vi "C-R Speed Test AIN eAddresses.vi"() -> ()   [LabVIEW 2020]
panel:
  in  "Case Constant\n(See Context Help)":bool
  out "Sorted Interval Array":ext[](array[numeric]) format="%.3g"
  in  "Range":dbl=10.0 format="%.2f"
  out "ConnectionType Out":i32
  out "DeviceType Out":i32
  in  "Identifier":string="LJM_idANY"
  in  "ConnectionType":string="LJM_ctANY"
  in  "DeviceType":string="LJM_dtANY"
  in  "Enable Interval Timing":bool
  out "min ms":ext format="%.3g"
  out "max ms":ext format="%.3g"
  out "avg ms per iteration":ext format="%.3f"
  out "Interval Array":ext[](array[numeric]) format="%.3g"
  in  "Write Both DACs":bool
  in  "Write Digital":bool
  in  "Read Digital":bool
  out "total ms":ext format="%.3g"
  in  "# Iterations":i32=1000
  in  "# AIN Channels":i32=1
  in  "Settling":i32
  out "Error Message":string
  in  "Resolution Index":i32=1
  out "error out":errorcluster
  # "Set controls as desired then click arrow (upper-left of window) to run.\n\nThis version uses a call before the loop to convert all names to addresses, and then inside the loop it uses a single call to eAddresses for all writes & reads."
  # "Interval timing uses the high resolution GetHostTick\nfunction from the LJM library."
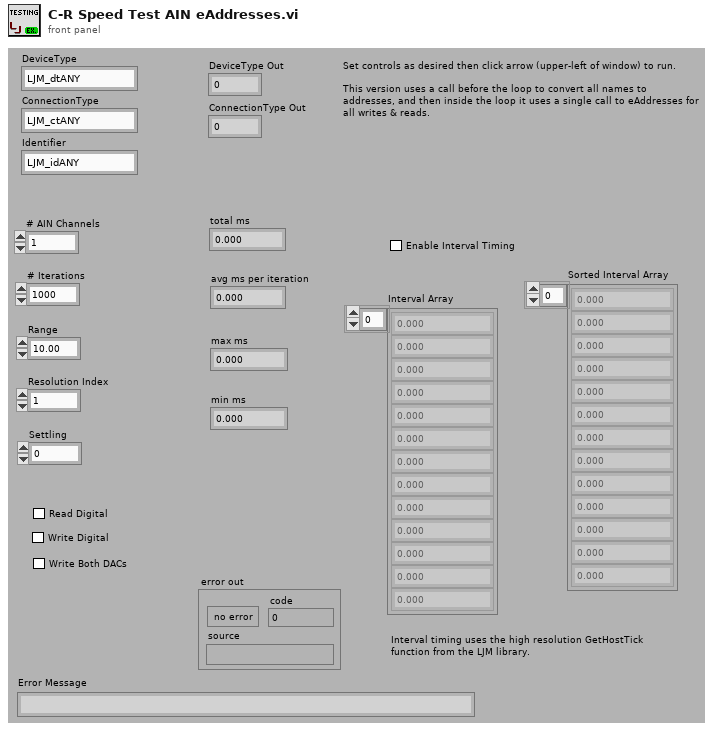
[diagram p1: front panel]
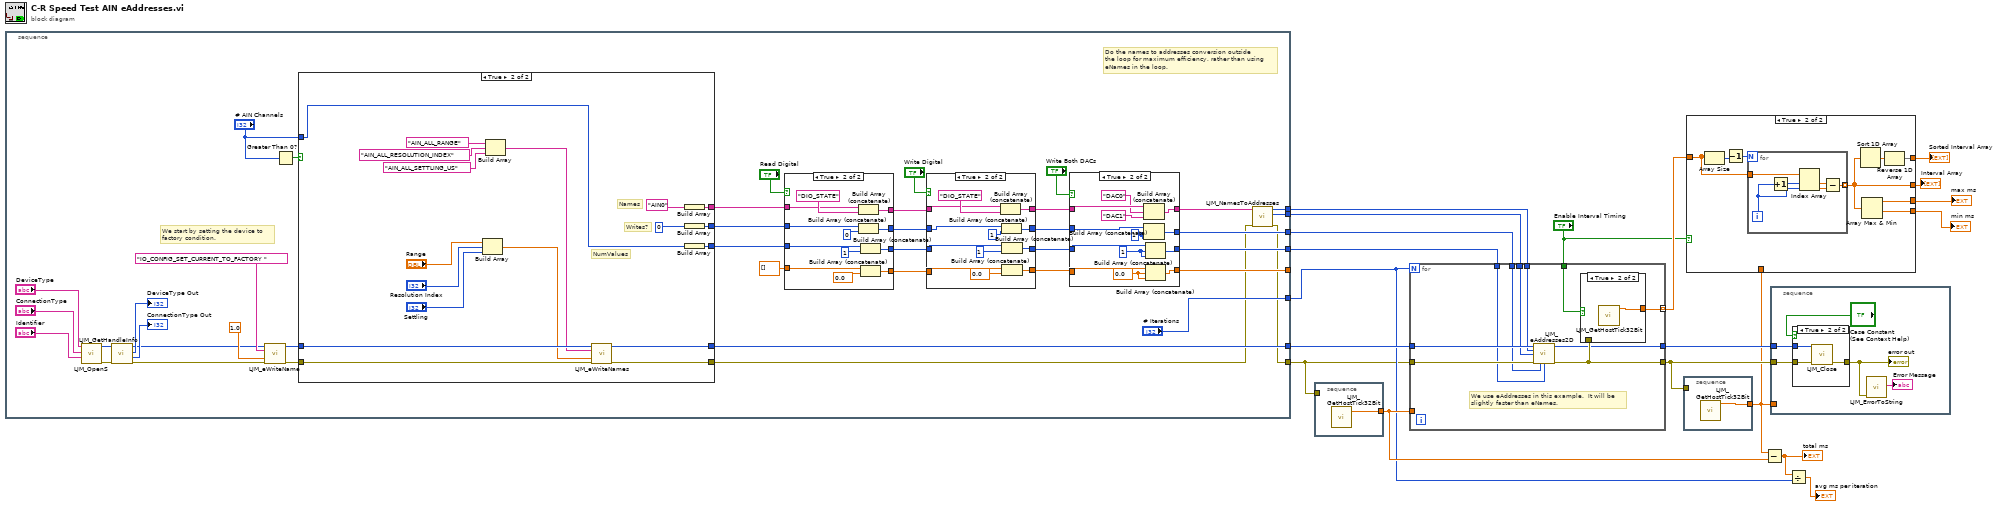
[diagram p0: block diagram]
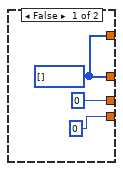
[diagram p2: hidden frame]
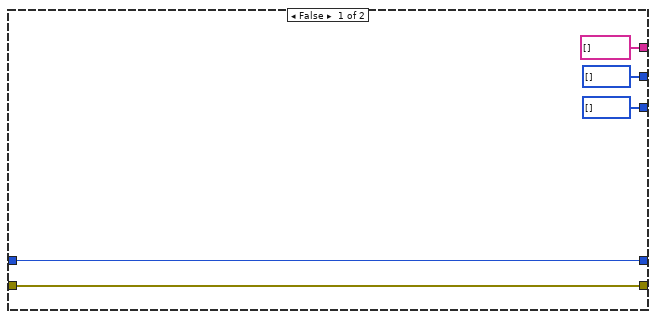
[diagram p4: hidden frame]
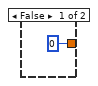
[diagram p8: hidden frame]
diagram:
  n1 = stacked-sequence {
    tunnel: [w40] -> w19
    tunnel: [w26] -> w2
    tunnel: ["# Iterations"] -> w14
    tunnel: [w29] -> w4
    tunnel: [w33] -> w10
    tunnel: [w32] -> w9
    tunnel: [w31] -> _
    tunnel: [w28] -> w3
    frame #0 {
      # "We start by setting the device to\nfactory condition."
      # "Do the names to addresses conversion outside\nthe loop for maximum efficiency, rather than using\neNames in the loop."
      n2 = call "LJM_OpenS.vi"("Identifier"="Identifier", "ConnectionType"="ConnectionType", "DeviceType"="DeviceType") -> ("error out"=w45:errorcluster, "Handle"=w46:i32)  [unwired: 7 in]
      n3 = call "LJM_GetHandleInfo.vi"("error in"=w45, "Handle In"=w46) -> ("error out"=w24:errorcluster, "ConnectionType"=→"ConnectionType Out":i32, "DeviceType"=→"DeviceType Out":i32, "Handle Out"=w21:i32)  [unwired: 2 in, 4 out]
      n4 = call "LJM_eWriteName.vi"("Handle In"=w21, "Name"="IO_CONFIG_SET_CURRENT_TO_FACTORY ", "Value"=1.0, "error in"=w24) -> ("Handle Out"=w20:i32, "error out"=w23:errorcluster)  [unwired: 10 in]
      n5 = Greater Than 0?(x="# AIN Channels") -> (x > 0?=w42:bool)
      n6 = case shown="True" w42 {
        tunnel: "# AIN Channels" -> [_ w72]
        tunnel: w20 -> [w64 w82]
        tunnel: w23 -> [w63 w81]
        tunnel: [w63 w80] -> w27
        tunnel: [w64 w79] -> w40
        tunnel: [string[] [] w74] -> w39
        tunnel: [i32[] [] w73] -> w38
        tunnel: [i32[] [] w71] -> w36
        frame False {
        }
        frame True {
          # "NumValues"
          # "Names"
          # "Writes?"
          n7 = Build Array("Range", "Resolution Index", "Settling") -> (w78:dbl[])
          n8 = Build Array("AIN_ALL_RANGE" ("Substring"), "AIN_ALL_RESOLUTION_INDEX" ("Substring"), "AIN_ALL_SETTLING_US" ("Substring")) -> (w77:string[])
          n9 = call "LJM_eWriteNames.vi"("Handle In"=w82, "aNames"=w77, "aValuesIn"=w78, "error in"=w81) -> ("Handle Out"=w79:i32, "error out"=w80:errorcluster)  [unwired: 9 in, 1 out]
          n10 = Build Array("AIN0") -> (w74:string[])
          n11 = Build Array(0) -> (w73:i32[])
          n12 = Build Array(w72) -> (w71:i32[])
        }
      }
      n13 = case shown="True" "Read Digital" {
        tunnel: [w119 w126] -> w57
        tunnel: [w117 w128] -> w56
        tunnel: [w116 w127] -> w55
        tunnel: w39 -> [w119 w125]
        tunnel: w38 -> [w118 w124]
        tunnel: dbl[] [] ("Input Array") -> [w116 w123]
        tunnel: w36 -> [w117 w122]
        tunnel: [w118 w121] -> w35
        frame False {
        }
        frame True {
          n14 = Build Array (concatenate)(w125, "DIO_STATE" ("IOType")) -> (w126:string[])
          n15 = Build Array (concatenate)(w124, 0) -> (w121:i32[])
          n16 = Build Array (concatenate)(w122, 1) -> (w128:i32[])
          n17 = Build Array (concatenate)(w123, 0.0) -> (w127:dbl[])
        }
      }
      n18 = case shown="True" "Write Digital" {
        tunnel: [w103 w115] -> w54
        tunnel: w57 -> [w103 w113]
        tunnel: [w102 w109] -> w53
        tunnel: w56 -> [w102 w112]
        tunnel: w55 -> [w101 w108]
        tunnel: [w101 w107] -> w52
        tunnel: w35 -> [w100 w106]
        tunnel: [w100 w104] -> w34
        frame False {
        }
        frame True {
          n19 = Build Array (concatenate)(w113, "DIO_STATE" ("IOType")) -> (w115:string[])
          n20 = Build Array (concatenate)(w106, 1) -> (w104:i32[])
          n21 = Build Array (concatenate)(w112, 1) -> (w109:i32[])
          n22 = Build Array (concatenate)(w108, 0.0) -> (w107:dbl[])
        }
      }
      n23 = case shown="True" "Write Both DACs" {
        tunnel: [w86 w99] -> w30
        tunnel: w54 -> [w86 w98]
        tunnel: [w85 w96] -> w32
        tunnel: w53 -> [w85 w97]
        tunnel: w52 -> [w84 w95]
        tunnel: [w84 w94] -> w31
        tunnel: w34 -> [w83 w88]
        tunnel: [w83 w87] -> w33
        frame False {
        }
        frame True {
          w89 = 1
          w92 = 0.0
          w93 = 1
          n24 = Build Array (concatenate)(w98, "DAC0" ("IOType"), "DAC1" ("Input Element")) -> (w99:string[])
          n25 = Build Array (concatenate)(w88, w89, w89) -> (w87:i32[])
          n26 = Build Array (concatenate)(w97, w93, w93) -> (w96:i32[])
          n27 = Build Array (concatenate)(w95, w92, w92) -> (w94:dbl[])
        }
      }
      n28 = call "LJM_NamesToAddresses.vi"("error in"=w27, "aNames"=w30) -> ("error out"=w26:errorcluster, "aTypes"=w28:i32[], "aAddresses"=w29:i32[])  [unwired: 7 in]
    }
  }
  n29 = stacked-sequence {
    tunnel: w2 -> [_]
    tunnel: [w132] -> w17
    frame #0 {
      n30 = call "LJM_GetHostTick32Bit.vi"() -> ("Tick Ext [ms]"=w132:ext)  [unwired: 9 in, 2 out]
    }
  }
  n31 = for {
    N: w14 -> [_]
    tunnel: w19 -> [w142]
    tunnel: w2 -> [w141]
    tunnel: [w139] -> w18
    tunnel: w17 -> [_]
    tunnel: "Enable Interval Timing" -> [w140]
    tunnel: [w138] -> w7 mode=indexing
    tunnel: w10 -> [w137]
    tunnel: w9 -> [w136]
    tunnel: [w135] -> w8
    tunnel: w3 -> [w134]
    tunnel: w4 -> [w133]
    # "We use eAddresses in this example.  It will be\nslightly faster than eNames."
    n32 = call "LJM_eAddresses2D.vi"("Handle In"=w142, "aAddresses"=w133, "aTypes"=w134, "error in"=w141, "aWrites"=w137, "aNumValues"=w136) -> ("Handle Out"=w135:i32, "error out"=w139:errorcluster)  [unwired: 6 in, 2 out]
    n33 = case shown="True" w140 {
      tunnel: w139 -> [_ _]
      tunnel: [u32 0 ("millisecond timer value") w144] -> w138
      frame False {
      }
      frame True {
        n34 = call "LJM_GetHostTick32Bit.vi"() -> ("Tick Ext [ms]"=w144:ext)  [unwired: 9 in, 2 out]
      }
    }
  }
  n35 = stacked-sequence {
    tunnel: w18 -> [_]
    tunnel: [w145] -> w5
    frame #0 {
      n36 = call "LJM_GetHostTick32Bit.vi"() -> ("Tick Ext [ms]"=w145:ext)  [unwired: 9 in, 2 out]
    }
  }
  n37 = case shown="True" "Enable Interval Timing" {
    tunnel: [w146 w151] -> w13
    tunnel: [u32 0 w154] -> w12
    tunnel: [u32 0 w153] -> w11
    tunnel: w7 -> [_ w152]
    tunnel: w5 -> [_ _]
    tunnel: [w146 w149] -> w1
    frame False {
      w146 = u32[] []
    }
    frame True {
      n38 = Array Size(array=w152) -> (size(s)=w156:i32)
      n39 = Decrement(x=w156) -> (x-1=w155:i32)
      n40 = for {
        N: w155 -> [_]
        tunnel: w152 -> [w162]
        tunnel: [w157] -> w151 mode=indexing
        i -> [w160]
        n41 = Increment(x=w160) -> (x+1=w161:i32)
        n42 = Index Array(array=w162, index #1=w161, index #2=w160) -> (element #1=w158:ext, element #2=w159:ext)
        n43 = Subtract(x=w158, y=w159) -> (x-y=w157:ext)
      }
      n44 = Sort 1D Array(array=w151) -> (sorted array=w150:ext[])
      n45 = Array Max & Min(array=w151) -> (max value=w154:ext, min value=w153:ext)  [unwired: 2 out]
      n46 = Reverse 1D Array(array=w150) -> (reversed array=w149:ext[])
    }
  }
  "Interval Array" <- w13
  "min ms" <- w11
  "max ms" <- w12
  "Sorted Interval Array" <- w1
  n47 = Subtract(x=w5, y=w17) -> (x-y=w15:ext)
  "total ms" <- w15
  n48 = stacked-sequence {
    tunnel: w18 -> [w166]
    tunnel: w5 -> [_]
    tunnel: w8 -> [w164]
    frame #0 {
      n49 = case shown="True" "Case Constant\n(See Context Help)" {
        tunnel: w166 -> [w168 w171]
        tunnel: [w168 w170] -> w165
        tunnel: w164 -> [_ w169]
        frame False {
        }
        frame True {
          n50 = call "LJM_Close.vi"("error in"=w171, "Handle"=w169) -> ("error out"=w170:errorcluster)  [unwired: 9 in]
        }
      }
      "error out" <- w165
      n51 = call "LJM_ErrorToString.vi"("error in"=w165) -> ("String"=→"Error Message":string)  [unwired: 10 in]
    }
  }
  n52 = Divide(x=w15, y=w14) -> (x/y=→"avg ms per iteration":ext)
